vi "PSTR-AO Thread.vi"(0 "Runtime":T1 {"window" items=["None ", "Hanning", "Hamming", "Blackman-Harris", "Exact Blackman", "Blackman", "Flat Top", "4 Term B-Harris ", "7 Term B-Harris", "Low Sidelobe"]}, 7 "abort":refnum<notifier>, 11 "error in (no error)":errorcluster) -> (15 "error out":errorcluster)   [LabVIEW 2020]
uses:
  Typedefs/PSTR-Runtime Data.ctl
  epl-vi-lib/Signal Synthesis VIs/4th Generation/Classes/SignalManager/SignalManager.lvclass
  epl-vi-lib/PXI DAQ VIs/AODO/Typedefs/AODO-Action.ctl
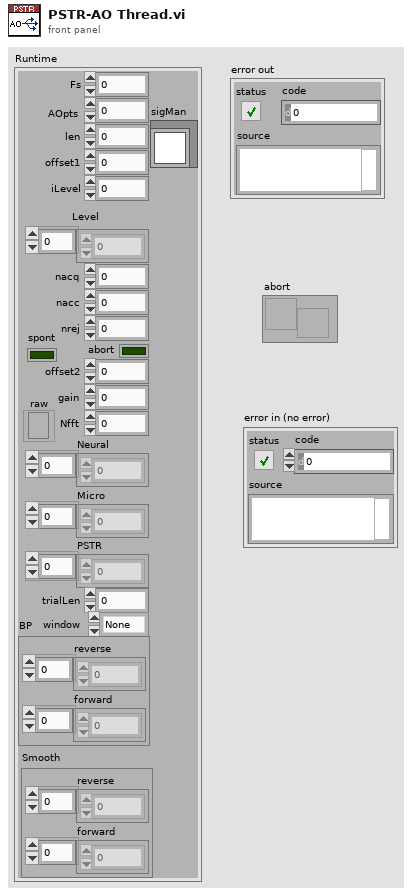
[diagram p1: front panel]
types:
  T1 = typedef "PSTR-Runtime Data.ctl" = cluster{"Fs":dbl, "AOpts":i32, "len":i32, "offset1":i32, "iLevel":i32, "Level":dbl[], "nacc":i32, "nrej":i32, "nacq":i32, "abort":bool, "offset2":i32, "gain":dbl, "Nfft":i32, "Neural":dbl[], "Micro":dbl[], "raw":refnum<file>, "spont":bool, "PSTR":dbl[], "trialLen":i32, "window":u16, "BP":cluster{"reverse":dbl[], "forward":dbl[]}, "Smooth":cluster{"reverse":dbl[], "forward":dbl[]}, "sigMan":refnum<class "SignalManager.lvclass">}
  T2 = typedef "AODO-Action.ctl" = enum16{"Configure", "Initialize", "Start", "Write", "Clean up", "Init & Start", "Config & Test", "Position", "Set AO Gains", "Zero", "Prime", "Status"}
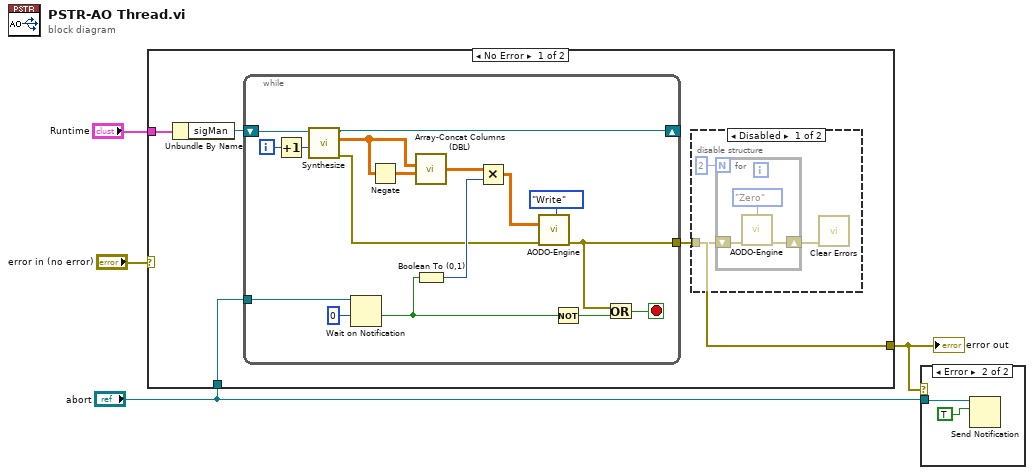
[diagram p0: block diagram]
diagram:
  n1 = case shown="No Error" "error in (no error)" {
    selector: "error in (no error)" -> [_ w32]
    tunnel: "abort" -> [w8 _]
    tunnel: [w7 w32] -> w3
    tunnel: "Runtime" -> [w6 _]
    frame No Error {
      n2 = Unbundle By Name(w6) -> ("sigMan"=w5:refnum<class "SignalManager.lvclass">)
      n3 = while {
        shift-right: [w22] -> _
        shift-left: w5 -> [w24]
        tunnel: [w26] -> w7
        tunnel: w8 -> [w31]
        i -> [w23]
        stop <- w27 stop-if-true
        n4 = Increment(x=w23) -> (x+1=w18:i32)
        n5 = call "Synthesize.vi"("Repetition"=w18, "SigMan in"=w24) -> ("error out"=w20:errorcluster, "Array"=w17:dbl[][], "SigMan out"=w22:refnum<class "SignalManager.lvclass">)  [unwired: 7 in]
        n6 = Wait on Notification(notifier=w31, timeout in ms (-1)=0) -> (timed out?=w29:bool)  [unwired: 2 in, 3 out]
        n7 = Negate(x=w17) -> (-x=w16:dbl[][])
        n8 = call "Array-Concat Columns (DBL).vi"("Array 2"=w16, "Array 1"=w17) -> ("concatenated array"=w15:dbl[][])  [unwired: 4 in]
        n9 = Boolean To (0,1)(Boolean=w29) -> (0, 1=w28:i16)
        n10 = Multiply(x=w15, y=w28) -> (x*y=w21:dbl[][])
        n11 = call "AODO-Engine.vi"("Action"=AODO-Action."Write", "AO"=w21, "error in (no error)"=w20) -> ("error out"=w26:errorcluster)  [unwired: 7 in, 5 out]
        n12 = Not(x=w29) -> (.not. x?=w25:bool)
        n13 = Or(x=w26, y=w25) -> (x .or. y?=w27:bool)
      }
      n14 = disable-structure shown="Disabled" {
        disable-tunnel: w7 -> [w10 _]
        frame Disabled {
          n15 = for {
            N: 2 -> [_]
            shift-right: [w12] -> w11
            shift-left: w10 -> [w13]
            n16 = call "AODO-Engine.vi"("Action"=AODO-Action."Zero", "error in (no error)"=w13) -> ("error out"=w12:errorcluster)  [unwired: 8 in, 5 out]
          }
          n17 = call <vilib>:"Clear Errors.vi"("error in (no error)"=w11) -> ()  [unwired: 5 in, 2 out]
        }
        frame Enabled {
        }
      }
    }
    frame Error {
    }
  }
  "error out" <- w3
  n18 = case shown="Error" w3 {
    tunnel: "abort" -> [_ w34]
    frame No Error {
    }
    frame Error {
      n19 = Send Notification(notification=TRUE, notifier=w34) -> ()  [unwired: 1 in, 2 out]
    }
  }
